vi "coagBuffer.vi"(4 "all coag in":dbl[](array[numeric]), 6 "command":T1=enum."read recent", 8 "error in (no error)":errorcluster, 10 "max array size":u16=5000 min=1, 11 "Coag dose":dbl) -> (0 "error out":errorcluster, 1 "all coag out":dbl[](array[numeric]), 3 "recent coag":dbl)   [LabVIEW 2019]
uses:
  ProCoDA/DAQ configuration/Sensor buffer command.ctl
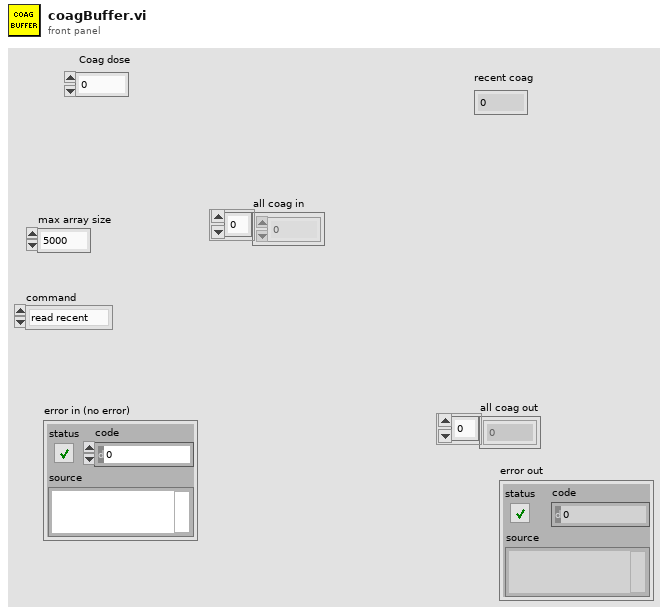
[diagram p1: front panel]
types:
  T1 = typedef "Sensor buffer command.ctl" = enum16{"set buffer size", "write", "refill buffer", "read recent", "read all", "clear"}
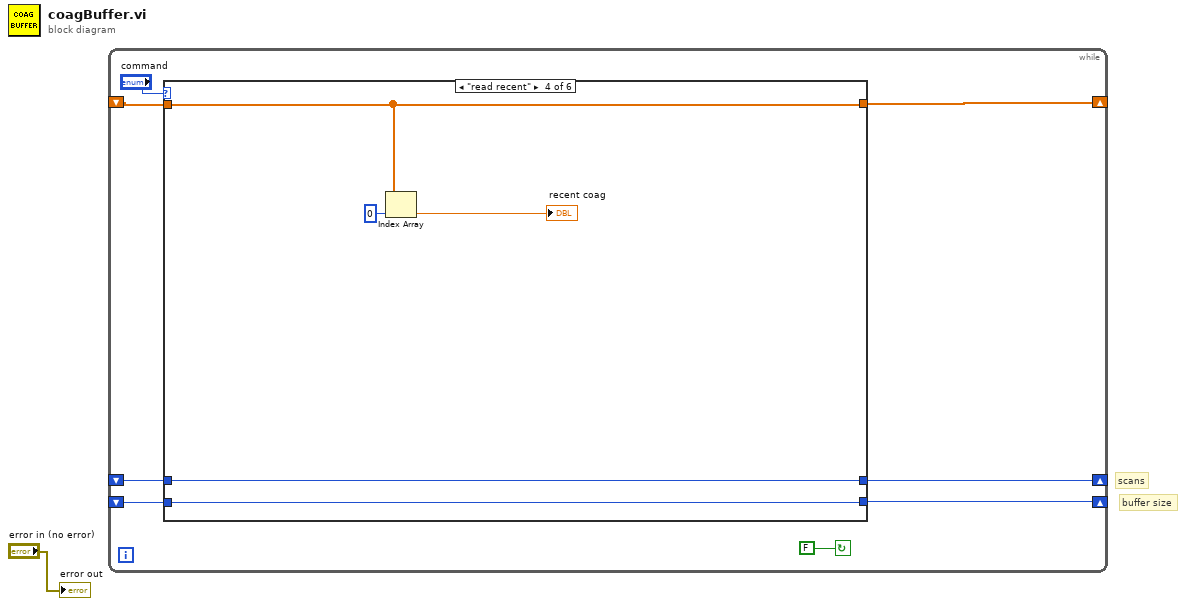
[diagram p0: block diagram]
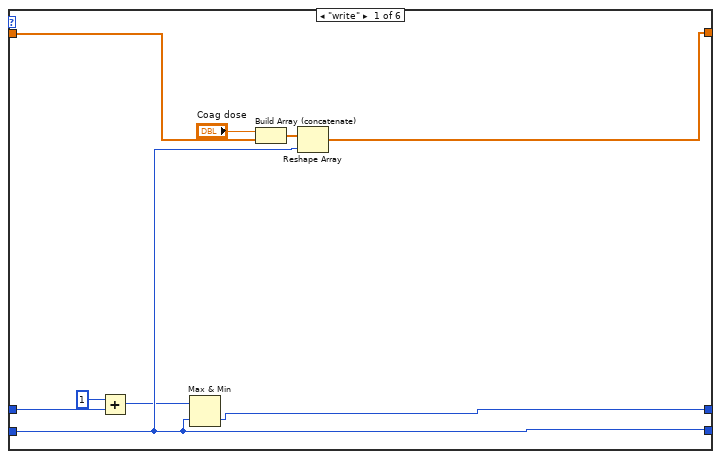
[diagram p2: hidden frame]
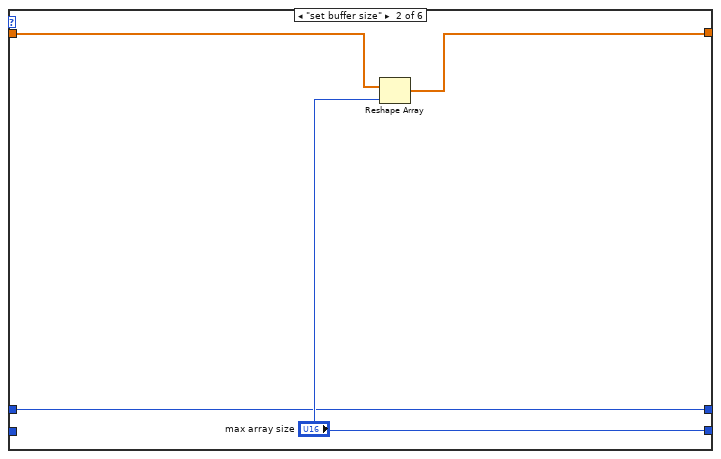
[diagram p3: hidden frame]
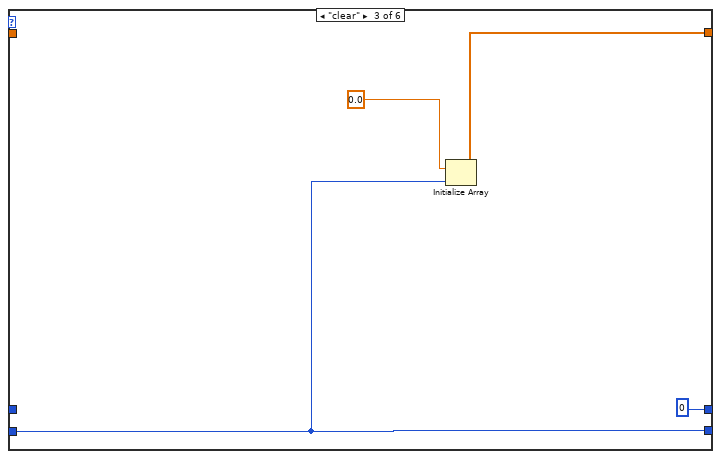
[diagram p4: hidden frame]
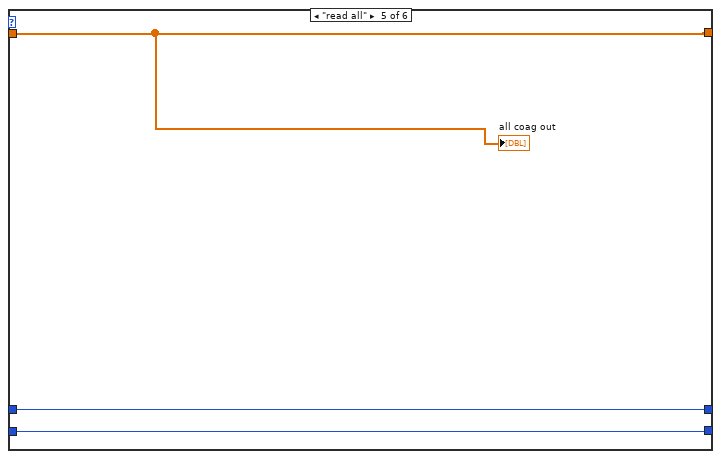
[diagram p5: hidden frame]
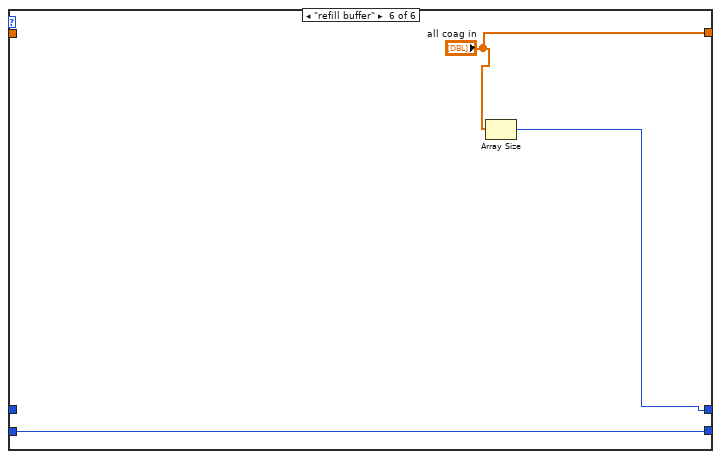
[diagram p6: hidden frame]
diagram:
  # "buffer size"
  # "scans"
  n1 = while {
    shift-right: [w8] -> _
    shift-left: _ -> [w7]
    shift-right: [w6] -> _
    shift-left: _ -> [w5]
    shift-right: [w2] -> _
    shift-left: _ -> [w3]
    stop <- FALSE continue-if-true
    n2 = case shown="\"read recent\"" "command" {
      tunnel: [w15 w21 w26 w31 w32 "all coag in"] -> w8
      tunnel: w7 -> [w17 w20 _ w31 w32 _]
      tunnel: [w13 "max array size" w25 w29 w34 w37] -> w6
      tunnel: w5 -> [w13 _ w25 w29 w34 w37]
      tunnel: w3 -> [w16 w19 _ w28 w33 _]
      tunnel: [w11 w19 0 w28 w33 w35] -> w2
      frame "write" {
        n3 = Add(x=1, y=w16) -> (x+y=w12:i32)
        n4 = Max & Min(x=w12, y=w13) -> (min(x,y)=w11:i32)  [unwired: 1 out]
        n5 = Build Array (concatenate)("Coag dose", w17) -> (w14:dbl[])
        n6 = Reshape Array(w14, w13) -> (w15:dbl[])
      }
      frame "set buffer size" {
        n7 = Reshape Array(w20, "max array size") -> (w21:dbl[])
      }
      frame "clear" {
        n8 = Initialize Array(0.0, w25) -> (w26:dbl[])
      }
      frame "read recent" {
        n9 = Index Array(array=w31, index=0) -> (element=→"recent coag":dbl)
      }
      frame "read all" {
        "all coag out" <- w32
      }
      frame "refill buffer" {
        n10 = Array Size(array="all coag in") -> (size(s)=w35:i32)
      }
    }
  }
  "error out" <- "error in (no error)"
